vi "Calibrate Sharp IR.vi"(10 "IR Raw In":dbl) -> (2 "IR Calibrated Out":dbl)   [LabVIEW 2014]
uses:
  <vilib>/ptbypt/NI_PtbyPt.lvlib
panel:
  # "This subVI calibrates the Sharp IR Range Sensors"
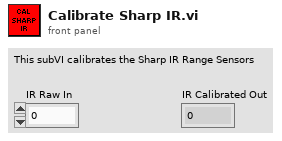
[diagram p1: front panel]
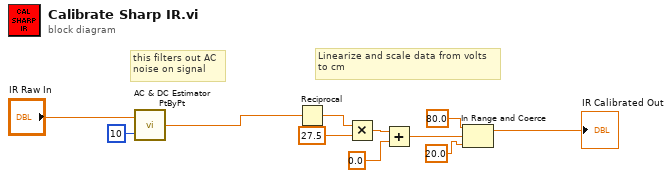
[diagram p0: block diagram]
diagram:
  # "Linearize and scale data from volts\nto cm"
  # "this filters out AC\nnoise on signal"
  n1 = call <vilib>:"AC & DC Estimator PtByPt.vi"("signal"="IR Raw In", "sample length"=10) -> ("DC estimate (V)"=w11:dbl)  [unwired: 1 in, 2 out]
  n2 = Reciprocal(x=w11) -> (1/x=w3:dbl)
  n3 = Multiply(x=w3, y=27.5 ("Kscale [cm-V]")) -> (x*y=w6:dbl)
  n4 = Add(x=w6, y=0.0 ("Koffset [cm]")) -> (x+y=w7:dbl)
  n5 = In Range and Coerce(upper limit=80.0, x=w7, lower limit=20.0) -> (coerced(x)=→"IR Calibrated Out":dbl)  [unwired: 1 out]
